vi "DPO_7K_Set_Channel_Position.vi"(8 "Error In":errorcluster, 9 "Position":dbl, 10 "Channel":u16(ring) items=["Channel 1", "Channel 2", "Channel 3", "Channel 4", "Math 1", "Math 2", "Math 3", "Math 4", "Reference 1", "Reference 2", "Reference 3", "Reference 4"], 11 "VISA resource name in":refnum<visa-resource-name>) -> (0 "Error Out":errorcluster, 3 "VISA resource name out":refnum<visa-resource-name>)   [LabVIEW 2020]
uses:
  subVI/Return_To_Interface.ctl
  subVI/Set_Configuration.ctl
panel:
  in  "Set":T1
  in  "Return to Interface":T2
  # "SET CHANNEL POSITION"
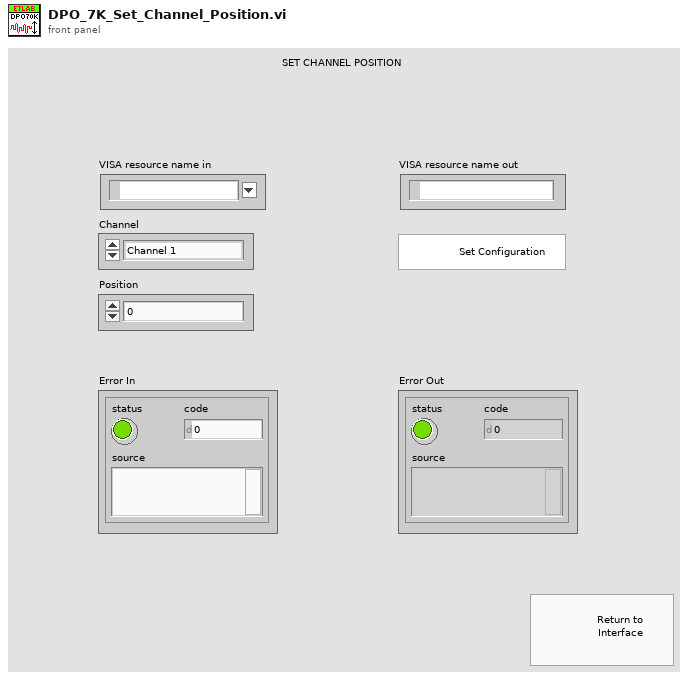
[diagram p1: front panel]
types:
  T1 = typedef "Set_Configuration.ctl" = bool
  T2 = typedef "Return_To_Interface.ctl" = bool
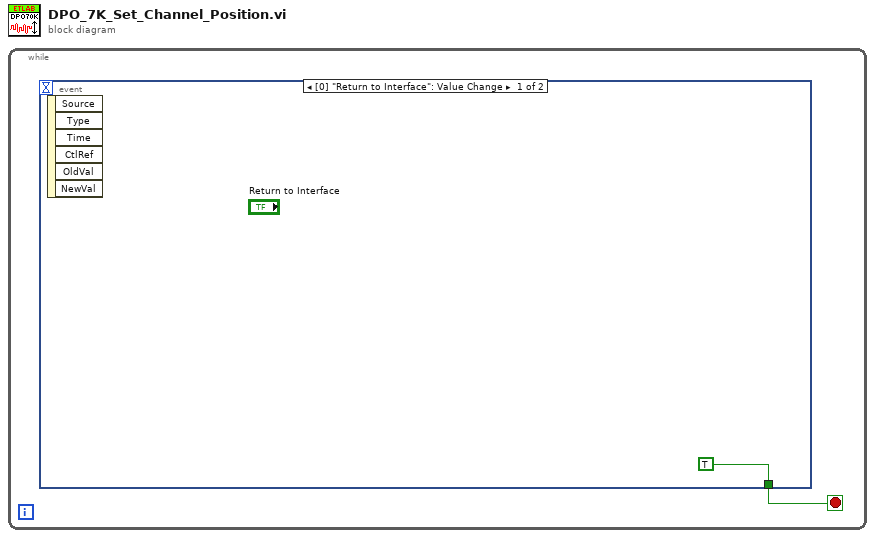
[diagram p0: block diagram]
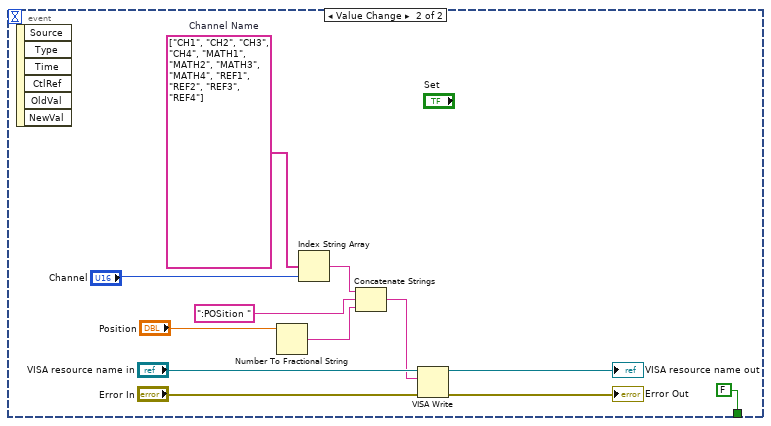
[diagram p2: hidden frame]
diagram:
  n1 = while {
    stop <- w1 stop-if-true
    n2 = event shown="[0] \"Return to Interface\": Value Change" {
      selector: _ -> [_ _]
      dyn-events: _ -> [_ _]
      timeout: _ -> [_ _]
      tunnel: [TRUE FALSE] -> w1
      event Value Change {
        n3 = event-data() -> ()  [unwired: 1 in, 6 out]
      }
      event Value Change {
        w5 = string[] ["CH1", "CH2", "CH3", "CH4", "MATH1", "MATH2", "MATH3", "MATH4", "REF1", "REF2", "REF3", "REF4"]  # Channel Name
        n4 = event-data() -> ()  [unwired: 1 in, 6 out]
        n5 = Number To Fractional String(number="Position") -> (F-format string=w10:string)  [unwired: 3 in]
        n6 = Index String Array(1:"Channel", 2:w5) -> (0:w7:string)  [unwired: 1 in]
        n7 = Concatenate Strings(w7, ":POSition " ("write buffer"), w10) -> (w6:string)
        n8 = VISA Write(VISA resource name="VISA resource name in", write buffer=w6, error in (no error)="Error In") -> (VISA resource name out=→"VISA resource name out":refnum<visa-resource-name>, error out=→"Error Out":errorcluster)  [unwired: 1 out]
      }
    }
  }
